vi "launchSubVI.vi"(0 "User Event in":refnum<user-event>, 5 "Boolean out":refnum<vi>, 7 "Path":path, 9 "Sub Panel":refnum<vi>) -> (4 "Sub Panel out":refnum<vi>, 8 "vi out":refnum<vi>)   [LabVIEW 2013]
uses:
  Controls/eventtypdef1.ctl
  Controls/GUI_cluster.ctl
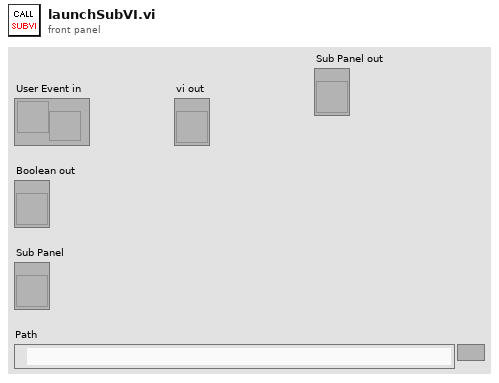
[diagram p1: front panel]
types:
  T1 = typedef "GUI_cluster.ctl" = cluster{"Sub Panel":refnum<vi>, "GUIdevice":string, "CtlRef":refnum<vi>, "User Event in":refnum<user-event>}
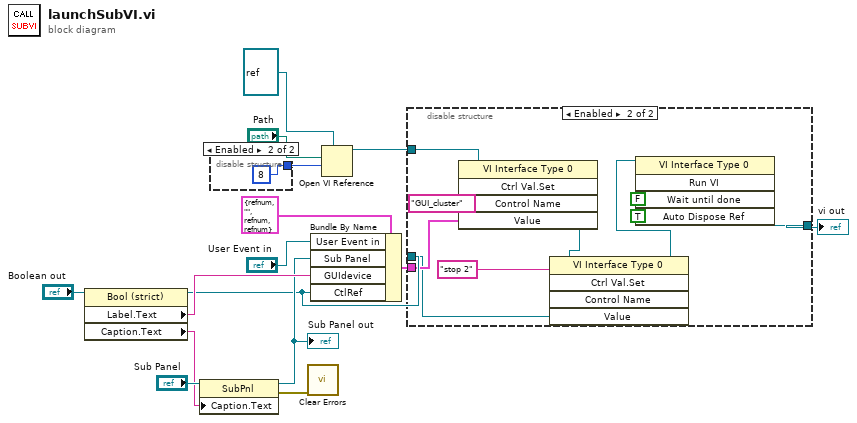
[diagram p0: block diagram]
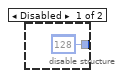
[diagram p2: hidden frame]
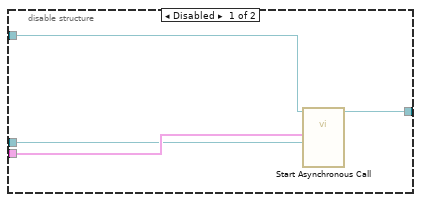
[diagram p3: hidden frame]
diagram:
  n1 = property class="Bool (strict)"(reference="Boolean out") -> (reference out=w2:refnum<vi>, "Label.Text"=w13:string, "Caption.Text"=w4:string)  [unwired: 1 in, 1 out]
  n2 = property class="SubPnl"(reference="Sub Panel", "Caption.Text"=w4) -> (reference out=w5:refnum<vi>, error out=w3:errorcluster)  [unwired: 1 in]
  "Sub Panel out" <- w5
  n3 = disable-structure shown="Enabled" {
    disable-tunnel: [128 ("options") 8 ("options")] -> w7
    frame Disabled {
      (unwired) 128 ("options")
    }
    frame Enabled {
    }
  }
  n4 = call <vilib>:"Clear Errors.vi"("error in (no error)"=w3) -> ()  [unwired: 6 in, 1 out]
  n5 = Bundle By Name(cluster=T1 {"Sub Panel"=refnum, "GUIdevice"="", "CtlRef"=refnum, "User Event in"=refnum} ("GUI_cluster"), "User Event in"="User Event in", "Sub Panel"=w5, "GUIdevice"=w13, "CtlRef"=w2) -> (w12:T1)
  n6 = Open VI Reference(type specifier VI Refnum (for type only)=refnum<vi> refnum, vi path="Path", options=w7) -> (vi reference=w10:refnum<vi>)  [unwired: 3 in, 1 out]
  n7 = disable-structure shown="Enabled" {
    disable-tunnel: w12 -> [w21 w26]
    disable-tunnel: w10 -> [w20 w27]
    disable-tunnel: w2 -> [w19 w24]
    disable-tunnel: [w18 w22] -> w1
    frame Disabled {
      n8 = call-by-ref "Start Asynchronous Call"(reference=w20, "stop 2"=w19, "GUI_cluster"=w21) -> (reference out=w18:refnum<vi>)  [unwired: 11 in, 1 out]
    }
    frame Enabled {
      n9 = invoke class="VI Interface Type 0" method="Ctrl Val.Set"(reference=w27, "Control Name"="GUI_cluster", "Value"=w26) -> (reference out=w31:refnum<vi>)  [unwired: 2 in, 4 out]
      n10 = invoke class="VI Interface Type 0" method="Ctrl Val.Set"(reference=w31, "Control Name"="stop 2", "Value"=w24) -> (reference out=w23:refnum<vi>)  [unwired: 2 in, 4 out]
      n11 = invoke class="VI Interface Type 0" method="Run VI"(reference=w23, "Wait until done"=FALSE ("Wait Until Done"), "Auto Dispose Ref"=TRUE ("Auto Dispose Reference")) -> (reference out=w22:refnum<vi>)  [unwired: 2 in, 4 out]
    }
  }
  "vi out" <- w1
